vi "LogTblParam (SubVI).vi"(8 "error in":errorcluster) -> (0 "error out":errorcluster)   [LabVIEW 2017]
uses:
  Global_SNK3_HF.vi
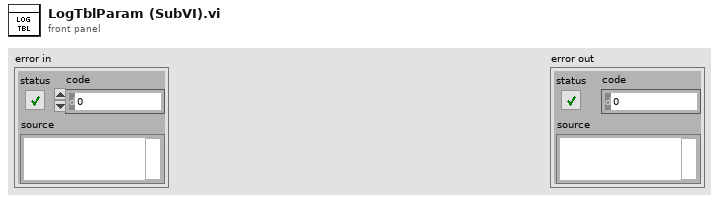
[diagram p1: front panel]
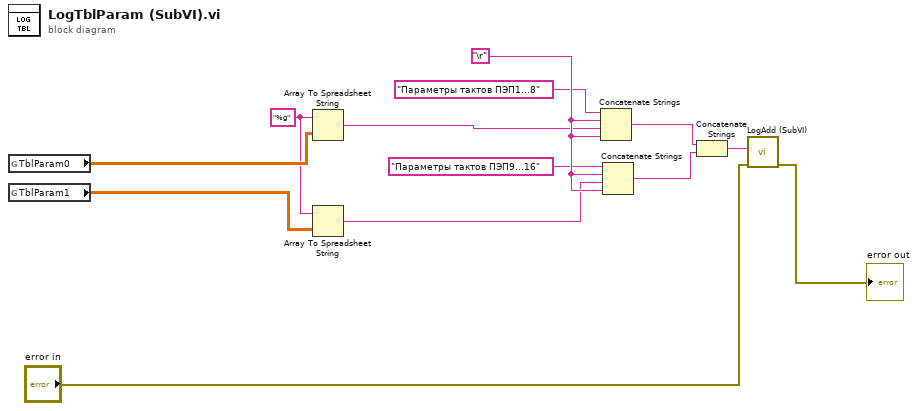
[diagram p0: block diagram]
diagram:
  w9 = "\r"
  w6 = "%g" ("format string")
  n1 = global read "Global_SNK3_HF.vi" "TblParam0"() -> (w13:sgl[][])
  n2 = global read "Global_SNK3_HF.vi" "TblParam1"() -> (w1:sgl[][])
  n3 = Array To Spreadsheet String(array=w13, 3:w6) -> (spreadsheet string=w7:string)  [unwired: 1 in]
  n4 = Array To Spreadsheet String(array=w1, 3:w6) -> (spreadsheet string=w8:string)  [unwired: 1 in]
  n5 = Concatenate Strings("Параметры тактов ПЭП1...8" ("string"), w9, w7, w9) -> (w10:string)
  n6 = Concatenate Strings("Параметры тактов ПЭП9...16" ("string"), w9, w8, w9) -> (w11:string)
  n7 = Concatenate Strings(w10, w11) -> (w12:string)
  n8 = call "LogAdd (SubVI).vi"("error in"="error in", "string"=w12) -> ("error out"=→"error out":errorcluster)  [unwired: 9 in]
